vi "Boxplot - Format Box Plots.vi"(6 "Plot Color":u32(colorbox)=16448250, 7 "XY Graph":refnum<vi>, 8 "error in (no error)":errorcluster, 11 "Number of Plots":i32) -> (0 "error out":errorcluster)   [LabVIEW 2023]
doc: "Formats all the parts of the boxplot."
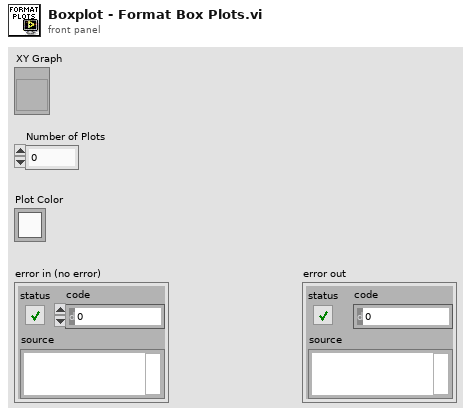
[diagram p1: front panel]
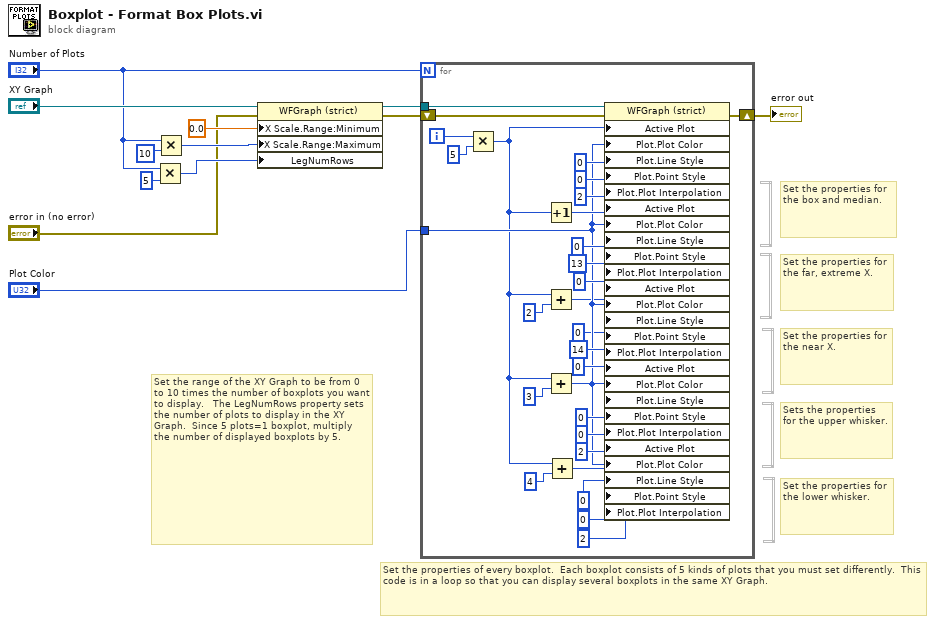
[diagram p0: block diagram]
diagram:
  # "Set the properties of every boxplot.  Each boxplot consists of 5 kinds of plots that you must set differently.  This code is in a loop so that you can display several boxplots in the same XY Graph."
  # "Set the range of the XY Graph to be from 0 to 10 times the number of boxplots you want to display.   The LegNumRows property sets the number of plots to display in the XY Graph.  Since 5 plots=1 boxplot, multiply the number of displayed boxplots by 5."
  # "Set the properties for the lower whisker."
  # "Sets the properties for the upper whisker."
  # "Set the properties for the near X."
  # "Set the properties for the far, extreme X."
  # "Set the properties for the box and median."
  n1 = Multiply(x="Number of Plots", y=5 ("Legend:Plots Shown")) -> (x*y=w12:i32)
  n2 = Multiply(x="Number of Plots", y=10 ("Legend:Plots Shown")) -> (x*y=w9:i32)
  n3 = property on="Property Node" class="WFGraph (strict)"(reference="XY Graph", error in="error in (no error)", "X Scale.Range:Minimum"=0.0 ("Legend:Plots Shown"), "X Scale.Range:Maximum"=w9, "LegNumRows"=w12) -> (reference out=w7:refnum<vi>, error out=w4:errorcluster)
  n4 = for {
    N: "Number of Plots" -> [_]
    tunnel: w7 -> [w41]
    shift-right: [w17] -> w3
    shift-left: w4 -> [w35]
    tunnel: "Plot Color" -> [w16]
    i -> [w38]
    n5 = Multiply(x=w38, y=5) -> (x*y=w13:i32)
    n6 = Increment(x=w13) -> (x+1=w34:i32)
    n7 = Add(x=w13, y=2) -> (x+y=w14:i32)
    n8 = Add(x=w13, y=3) -> (x+y=w26:i32)
    n9 = Add(x=w13, y=4) -> (x+y=w21:i32)
    n10 = property on="Property Node" class="WFGraph (strict)"(reference=w41, error in=w35, "Active Plot"=w13, "Plot.Plot Color"=w16, "Plot.Line Style"=u8 0, "Plot.Point Style"=u8 0, "Plot.Plot Interpolation"=u8 2, "Active Plot"=w34, "Plot.Plot Color"=w16, "Plot.Line Style"=u8 0 ("Plot.Line Style 2"), "Plot.Point Style"=u8 13 ("Plot.Point Style 2"), "Plot.Plot Interpolation"=u32 0 ("Active Cursor"), "Active Plot"=w14, "Plot.Plot Color"=w16, "Plot.Line Style"=u8 0 ("Plot.Line Style 3"), "Plot.Point Style"=u8 14 ("Plot.Point Style 3"), "Plot.Plot Interpolation"=u8 0, "Active Plot"=w26, "Plot.Plot Color"=w16, "Plot.Line Style"=u8 0 ("Plot.Line Style 4"), "Plot.Point Style"=u8 0 ("Plot.Point Style 4"), "Plot.Plot Interpolation"=u8 2, "Active Plot"=w21, "Plot.Plot Color"=w16, "Plot.Line Style"=u8 0 ("Plot.Line Style 5"), "Plot.Point Style"=u8 0 ("Plot.Point Style 5"), "Plot.Plot Interpolation"=u8 2) -> (error out=w17:errorcluster)  [unwired: 1 out]
  }
  "error out" <- w3
